vi "SetupDefault.vi"(8 "error in (no error)":errorcluster, 10 "Alias":string, 11 "PwrMtr_U2k in":refnum<class "PwrMtr_U2k.lvclass">) -> (0 "error out":errorcluster, 3 "PwrMtr_U2k out":refnum<class "PwrMtr_U2k.lvclass">)   [LabVIEW 2014, in "PwrMtr_U2k.lvclass"]
uses:
  PwrMtr_U2k.lvclass
  PwrMtr_U2k.lvclass/PwrMtr_U2k.ctl
  <instrlib>/Agilent U2000 Series/Agilent U2000 Series.lvlib
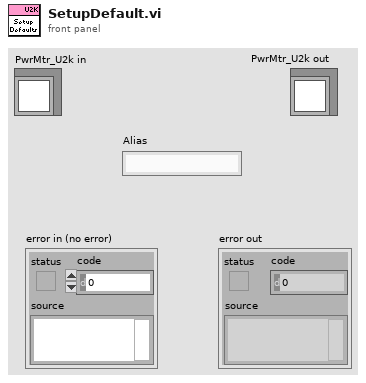
[diagram p1: front panel]
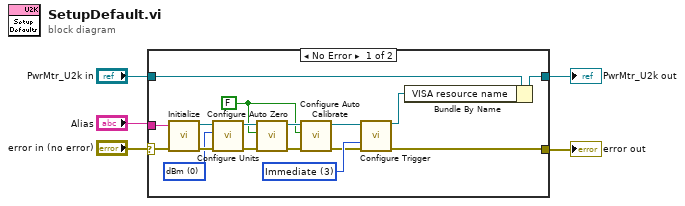
[diagram p0: block diagram]
diagram:
  n1 = case shown="No Error" "error in (no error)" {
    selector: "error in (no error)" -> [w16 w23]
    tunnel: "PwrMtr_U2k in" -> [w22 w24]
    tunnel: [w21 w24] -> w4
    tunnel: [w7 w23] -> w5
    tunnel: "Alias" -> [w8 _]
    frame No Error {
      w17 = u16 0 items=["dBm", "W"] ("Units")
      w9 = FALSE ("Auto Zero (T: Enable)")
      w18 = 3 items=["Bus", "External", "Hold", "Immediate", "Internal A"] ("Trigger Source (3: Immediate)")
      n2 = call <instrlib>:"Initialize.vi"("error in (no error)"=w16, "VISA resource name"=w8) -> ("error out"=w20:errorcluster, "VISA resource name out"=w19:refnum<visa-resource-name>)  [unwired: 2 in, 6 out]
      n3 = call <instrlib>:"Configure Units.vi"("error in (no error)"=w20, "Units (0: dBm)"=w17, "VISA resource name"=w19) -> ("error out"=w15:errorcluster, "VISA resource name out"=w14:refnum<visa-resource-name>)  [unwired: 1 in, 6 out]
      n4 = call <instrlib>:"Configure Auto Zero.vi"("error in (no error)"=w15, "Auto Zero (T: Enable)"=w9, "VISA resource name"=w14) -> ("error out"=w11:errorcluster, "VISA resource name out"=w13:refnum<visa-resource-name>)  [unwired: 7 in]
      n5 = call <instrlib>:"Configure Auto Calibrate.vi"("error in (no error)"=w11, "Auto Calibrate (T: Enable)"=w9, "VISA resource name"=w13) -> ("error out"=w10:errorcluster, "VISA resource name out"=w12:refnum<visa-resource-name>)  [unwired: 7 in]
      n6 = call <instrlib>:"Configure Trigger.vi"("VISA resource name"=w12, "Trigger Source (3: Immediate)"=w18, "error in (no error)"=w10) -> ("VISA resource name out"=w6:refnum<visa-resource-name>, "error out"=w7:errorcluster)  [unwired: 11 in]
      n7 = Bundle By Name(cluster=w22, "VISA resource name"=w6) -> (w21:refnum<class "PwrMtr_U2k.lvclass">)
    }
    frame Error {
    }
  }
  "error out" <- w5
  "PwrMtr_U2k out" <- w4
